vi "filter.clz_series.vi"(9 "filter char":string, 11 "clz series map":T1(c390)) -> (1 "series array":string[](array[string]), 3 "series map out":map{string, i32}(c390))   [LabVIEW 2024]
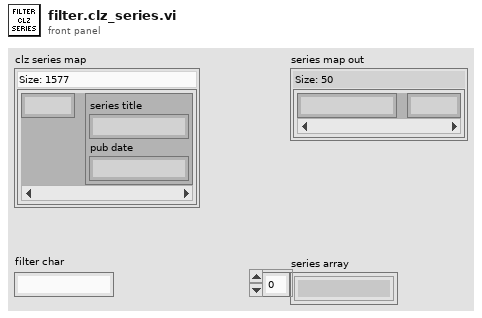
[diagram p1: front panel]
types:
  T1 = map{i32, cluster{"series title":string, "pub date":string}}
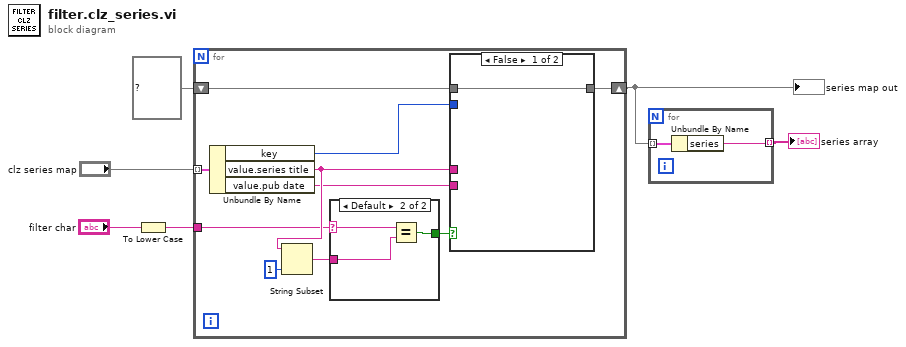
[diagram p0: block diagram]
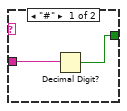
[diagram p2: hidden frame]
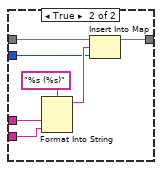
[diagram p3: hidden frame]
diagram:
  n1 = To Lower Case(string="filter char") -> (all lower case string=w6:string)
  n2 = for {
    tunnel: "clz series map" -> [w16] mode=indexing
    tunnel: w6 -> [w12]
    shift-right: [w7] -> w3
    shift-left: map{string, i32} {} ("map") -> [w9]
    n3 = Unbundle By Name(w16) -> ("key"=w8:i32, "value.series title"=w14:string, "value.pub date"=w13:string)
    n4 = String Subset(string=w14, length (rest)=1 ("offset (0)")) -> (substring=w10:string)  [unwired: 1 in]
    n5 = case shown="Default" w12 {
      selector: w12 -> [_ w20]
      tunnel: [w17 w21] -> w15
      tunnel: w10 -> [w18 w19]
      frame "#" {
        n6 = Decimal Digit?(1:w18) -> (0:w17:bool)
      }
      frame Default {
        n7 = Equal?(x=w20, y=w19) -> (x = y?=w21:bool)
      }
    }
    n8 = case shown="False" w15 {
      tunnel: w14 -> [_ w29]
      tunnel: w13 -> [_ w28]
      tunnel: w9 -> [w22 w26]
      tunnel: w8 -> [_ w24]
      tunnel: [w22 w23] -> w7
      frame False {
      }
      frame True {
        n9 = Format Into String(format string="%s (%s)", w29, w28) -> (resulting string=w25:string)  [unwired: 2 in, 1 out]
        n10 = Insert Into Map(map in=w26, key=w25, value=w24) -> (map out=w23:map{string, i32})  [unwired: 2 out]
      }
    }
  }
  "series map out" <- w3
  n11 = for {
    tunnel: w3 -> [w31] mode=indexing
    tunnel: [w30] -> w2 mode=indexing
    n12 = Unbundle By Name(w31) -> ("series"=w30:string)
  }
  "series array" <- w2
